vi "Read Accelerometer.vi"(5 "gyro range (deg/sec)":u16(ring)=250 items=["250"=250, "500"=500, "1000"=1000, "2000"=2000], 6 "retries":u16=5, 7 "accel range (g)":u16(ring)=2 items=["2"=2, "4"=4, "8"=8, "16"=16], 8 "error in (no error)":errorcluster, 9 "check ready":bool=TRUE, 11 "Accelerometer":T2) -> (0 "error out":errorcluster, 2 "Accelerometer Data":T1, 3 "Accelerometer out":T2, 4 "num tries":i32)   [LabVIEW 2013]
doc: "Use this template to build a VI to use as a subVI."
uses:
  Accelerometer.ctl
  <vilib>/ni845x/ni845x.llb/ni845xControl.ctl
  <vilib>/ni845x/ni845x.llb/ni845xI2cConfiguration.ctl
  Accelerometer Data.ctl
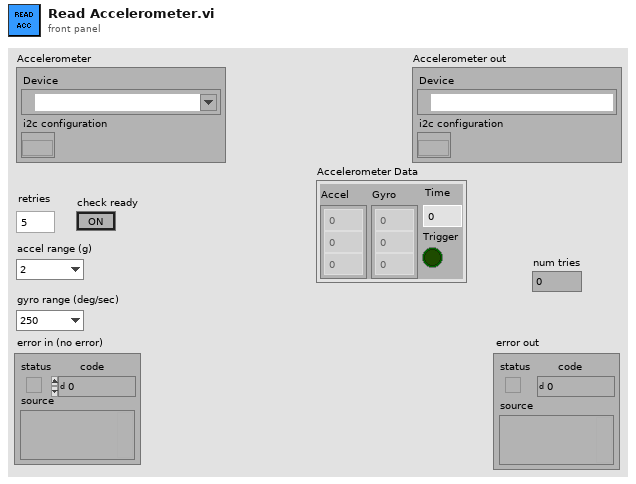
[diagram p1: front panel]
types:
  T1 = typedef "Accelerometer Data.ctl" = cluster{"Accel":dbl[], "Gyro":dbl[], "Time":u64, "Trigger":bool}
  T2 = typedef "Accelerometer.ctl" = cluster{"Device":T3, "i2c configuration":T4}
  T3 = typedef "ni845xControl.ctl" = refnum<k21>
  T4 = typedef "ni845xI2cConfiguration.ctl" = refnum<k20>
  T5 = typedef "ni845xDioLineWriteValue.ctl" = i32
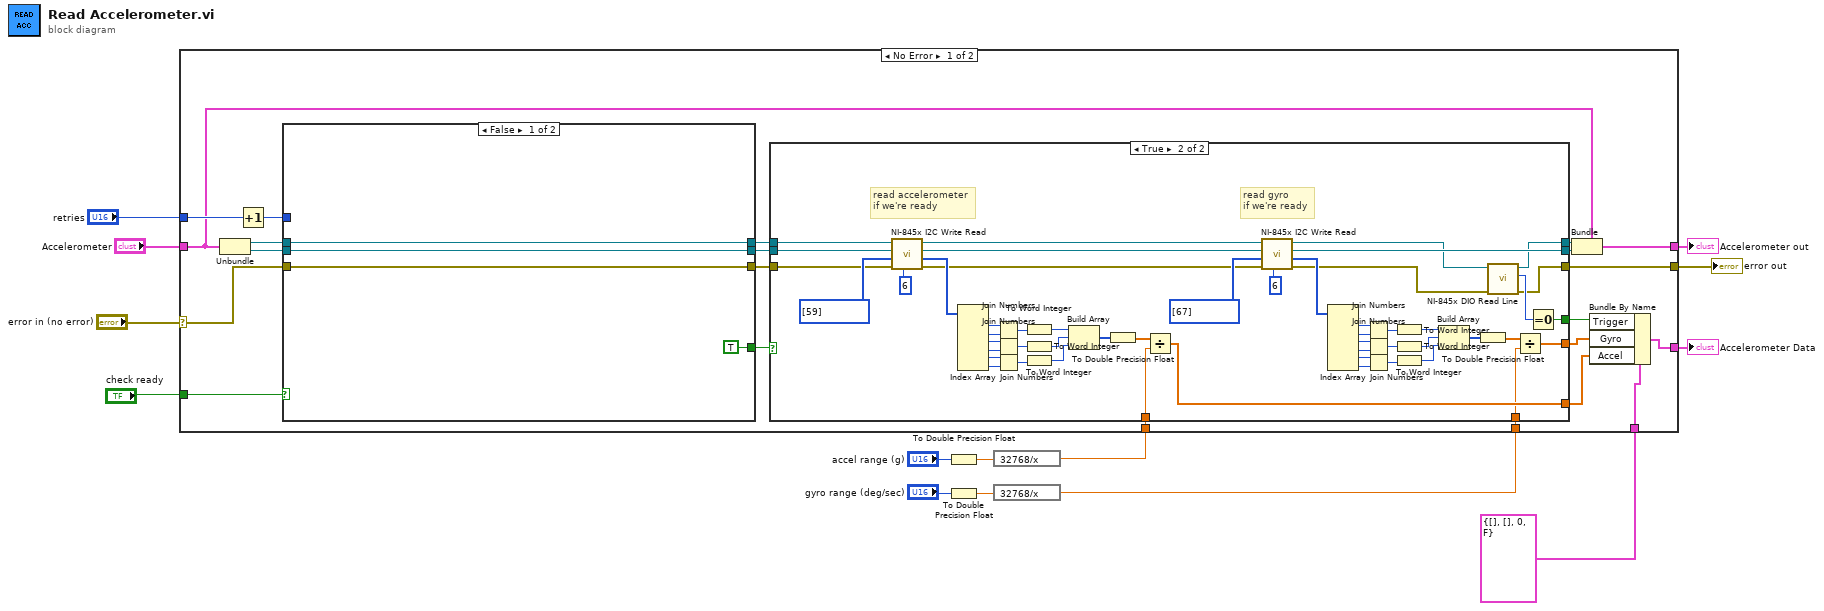
[diagram p0: block diagram]
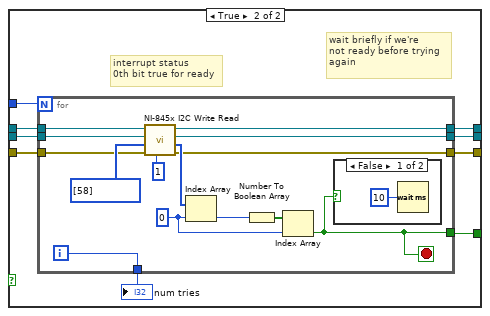
[diagram p2: hidden frame]
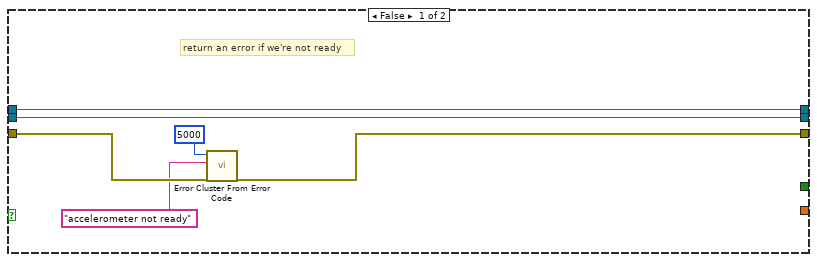
[diagram p4: hidden frame]
diagram:
  n1 = To Double Precision Float(number="accel range (g)") -> (double precision float=w7:dbl)
  n2 = To Double Precision Float(number="gyro range (deg/sec)") -> (double precision float=w6:dbl)
  n3 = expression code="32768/x"(w7) -> (w10:dbl)
  n4 = expression code="32768/x"(w6) -> (w5:dbl)
  n5 = case shown="No Error" "error in (no error)" {
    selector: "error in (no error)" -> [w32 w123]
    tunnel: [w35 w123] -> w13
    tunnel: "Accelerometer" -> [w22 w122]
    tunnel: [w23 w122] -> w11
    tunnel: w10 -> [w36 _]
    tunnel: "retries" -> [w30 _]
    tunnel: w5 -> [w21 _]
    tunnel: T1 {"Accel"=[], "Gyro"=[], "Time"=0, "Trigger"=FALSE} ("Accelerometer Data") -> [w20 _]
    tunnel: [w17 _] -> w2
    tunnel: "check ready" -> [w15 _]
    frame No Error {
      n6 = Unbundle(w22) -> ("Device"=w34:T3, "i2c configuration"=w33:T4)
      n7 = Increment(x=w30) -> (x+1=w31:u16)
      n8 = case shown="False" w15 {
        tunnel: w34 -> [w40 w49]
        tunnel: w33 -> [w39 w48]
        tunnel: w32 -> [w38 w47]
        tunnel: w31 -> [_ w46]
        tunnel: [TRUE w45] -> w29
        tunnel: [w38 w44] -> w28
        tunnel: [w40 w43] -> w27
        tunnel: [w39 w42] -> w26
        frame False {
        }
        frame True {
          # "wait briefly if we're\nnot ready before trying\nagain"
          # "interrupt status\n0th bit true for ready"
          n9 = for {
            N: w46 -> [_]
            tunnel: w49 -> [w61]
            tunnel: w48 -> [w60]
            tunnel: [w51] -> w45
            tunnel: [w55] -> w43
            tunnel: [w54] -> w42
            tunnel: [w53] -> w44
            tunnel: w47 -> [w52]
            tunnel: [w50] -> w41
            i -> [w50]
            stop <- w51 stop-if-true
            w56 = 0 ("index")
            n10 = call <vilib>:"NI-845x I2C Write Read.vi"("num bytes to read"=u32 1, "error in (no error)"=w52, "write data"=u8[] [58], "i2c configuration in"=w60, "device reference in"=w61) -> ("error out"=w53:errorcluster, "read data"=w59:u8[], "i2c configuration out"=w54:T4, "device reference out"=w55:T3)  [unwired: 3 in]
            n11 = Index Array(array=w59, index=w56) -> (element=w58:u8)
            n12 = Number To Boolean Array(number=w58) -> (Boolean array=w57:bool[])
            n13 = Index Array(array=w57, index=w56) -> (element=w51:bool)
            n14 = case shown="False" w51 {
              frame False {
                n15 = Wait (ms)(milliseconds to wait=u32 10) -> ()  [unwired: 1 out]
              }
              frame True {
              }
            }
          }
          "num tries" <- w41
        }
      }
      n16 = case shown="True" w29 {
        tunnel: w36 -> [_ w108]
        tunnel: [_ w100] -> w18
        tunnel: [w67 w73] -> w35
        tunnel: w28 -> [w70 w105]
        tunnel: w27 -> [w66 w107]
        tunnel: w26 -> [w65 w106]
        tunnel: [w66 w72] -> w25
        tunnel: [w65 w78] -> w24
        tunnel: w21 -> [_ w79]
        tunnel: [_ w77] -> w19
        tunnel: [_ w71] -> w16
        frame False {
          # "return an error if we're not ready"
          n17 = call <vilib>:"Error Cluster From Error Code.vi"("error in (no error)"=w70, "error message (\"\")"="accelerometer not ready" ("error message (\"\")"), "error code (0)"=5000) -> ("error out"=w67:errorcluster)  [unwired: 6 in]
        }
        frame True {
          # "read gyro\nif we're ready"
          # "read accelerometer\nif we're ready"
          n18 = call <vilib>:"NI-845x I2C Write Read.vi"("num bytes to read"=u32 6, "error in (no error)"=w105, "write data"=u8[] [59], "i2c configuration in"=w106, "device reference in"=w107) -> ("error out"=w80:errorcluster, "read data"=w119:u8[], "i2c configuration out"=w81:T4, "device reference out"=w82:T3)  [unwired: 3 in]
          n19 = Index Array(array=w119) -> (element #1=w117:u8, element #2=w118:u8, element #3=w114:u8, element #4=w116:u8, element #5=w113:u8, element #6=w115:u8)  [unwired: 6 in]
          n20 = Join Numbers(hi=w117, lo=w118) -> ((hi.lo)=w111:u16)
          n21 = Join Numbers(hi=w114, lo=w116) -> ((hi.lo)=w110:u16)
          n22 = Join Numbers(hi=w113, lo=w115) -> ((hi.lo)=w109:u16)
          n23 = To Word Integer(number=w111) -> (16bit integer=w104:i16)
          n24 = To Word Integer(number=w110) -> (16bit integer=w103:i16)
          n25 = To Word Integer(number=w109) -> (16bit integer=w102:i16)
          n26 = Build Array(w104, w103, w102) -> (w101:i16[])
          n27 = To Double Precision Float(number=w101) -> (double precision float=w112:dbl[])
          n28 = Divide(x=w112, y=w108) -> (x/y=w100:dbl[])
          n29 = call <vilib>:"NI-845x I2C Write Read.vi"("num bytes to read"=u32 6, "error in (no error)"=w80, "write data"=u8[] [67], "i2c configuration in"=w81, "device reference in"=w82) -> ("error out"=w75:errorcluster, "read data"=w85:u8[], "i2c configuration out"=w78:T4, "device reference out"=w76:T3)  [unwired: 3 in]
          n30 = Index Array(array=w85) -> (element #1=w87:u8, element #2=w86:u8, element #3=w90:u8, element #4=w88:u8, element #5=w91:u8, element #6=w89:u8)  [unwired: 6 in]
          n31 = Join Numbers(hi=w87, lo=w86) -> ((hi.lo)=w93:u16)
          n32 = Join Numbers(hi=w90, lo=w88) -> ((hi.lo)=w94:u16)
          n33 = Join Numbers(hi=w91, lo=w89) -> ((hi.lo)=w95:u16)
          n34 = To Word Integer(number=w93) -> (16bit integer=w96:i16)
          n35 = To Word Integer(number=w94) -> (16bit integer=w97:i16)
          n36 = To Word Integer(number=w95) -> (16bit integer=w98:i16)
          n37 = Build Array(w96, w97, w98) -> (w99:i16[])
          n38 = To Double Precision Float(number=w99) -> (double precision float=w92:dbl[])
          n39 = call <vilib>:"NI-845x DIO Read Line.vi"("error in (no error)"=w75, "device reference in"=w76) -> ("error out"=w73:errorcluster, "read value"=w74:T5, "device reference out"=w72:T3)  [unwired: 7 in]
          n40 = Divide(x=w92, y=w79) -> (x/y=w77:dbl[])
          n41 = Equal To 0?(x=w74) -> (x = 0?=w71:bool)
        }
      }
      n42 = Bundle(cluster=w22, "Device"=w25, "i2c configuration"=w24) -> (w23:T2)
      n43 = Bundle By Name(cluster=w20, "Trigger"=w16, "Gyro"=w19, "Accel"=w18) -> (w17:T1)
    }
    frame Error {
    }
  }
  "error out" <- w13
  "Accelerometer out" <- w11
  "Accelerometer Data" <- w2
